vi "Configure VCO Clock.vi"(8 "error in (no error)":errorcluster, 9 "VCO Clock Source (0: Internal)":u16(ring) items=["Internal", "External"], 10 "Modulation Format (0: Custom)":u16(ring) items=["Custom"=0, "Dual ARB"=2], 11 "VISA resource name":refnum<visa-resource-name>) -> (0 "error out":errorcluster, 3 "VISA resource name out":refnum<visa-resource-name>)   [LabVIEW 2018, in "Agilent PSG MXG Series.lvlib"]
doc: "Configures VCO clock source.\n\n<B>Notes:</B>\n(1) This VI is valid only in E8267D that installs <B>Option 601</B> or <B>Option 602</B> (Internal baseband generator)."
uses:
  Agilent PSG MXG Series.lvlib
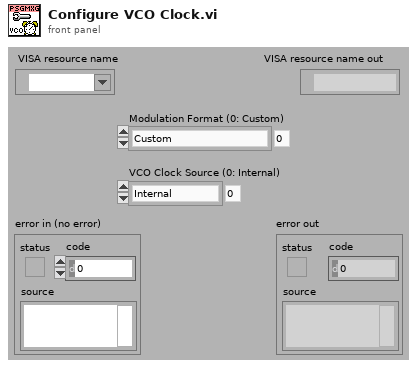
[diagram p1: front panel]
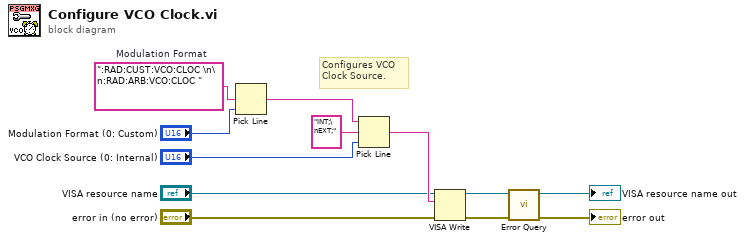
[diagram p0: block diagram]
diagram:
  w12 = ":RAD:CUST:VCO:CLOC \n\n:RAD:ARB:VCO:CLOC "  # Modulation Format
  # "Configures VCO\nClock Source."
  n1 = Pick Line(multi-line string=w12, line index="Modulation Format (0: Custom)") -> (output string=w10:string)  [unwired: 1 out]
  n2 = Pick Line(string ("")=w10, multi-line string="INT;\nEXT;", line index="VCO Clock Source (0: Internal)") -> (output string=w7:string)
  n3 = VISA Write(VISA resource name="VISA resource name", write buffer=w7, error in (no error)="error in (no error)") -> (VISA resource name out=w6:refnum<visa-resource-name>, error out=w5:errorcluster)  [unwired: 1 out]
  n4 = call "Error Query.vi"("error in (no error)"=w5, "VISA resource name"=w6) -> ("error out"=→"error out":errorcluster, "VISA resource name out"=→"VISA resource name out":refnum<visa-resource-name>)  [unwired: 8 out]
